vi "Shift.vi"(4 "Step count":i32, 5 "Step time (in ms)":u32, 6 "Absolute position":u16(ring) items=["Number of steps", "Absolute position"], 7 "Step size":i32, 8 "error in (no error)":errorcluster, 9 "Final position":i32, 10 "Movement direction":u16(ring) items=["Down", "Up", "Right", "Left"], 11 "Control in":refnum<vi>) -> (0 "error out":errorcluster, 3 "Current position":i32)   [LabVIEW 2019]
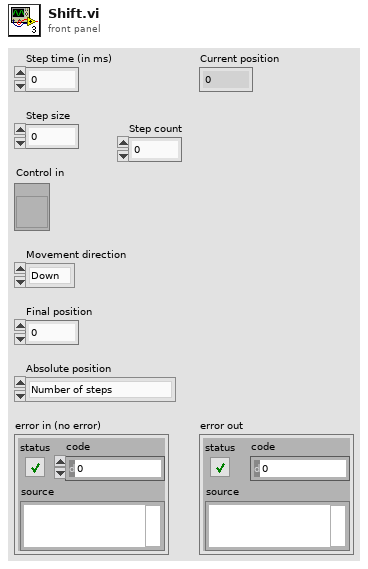
[diagram p1: front panel]
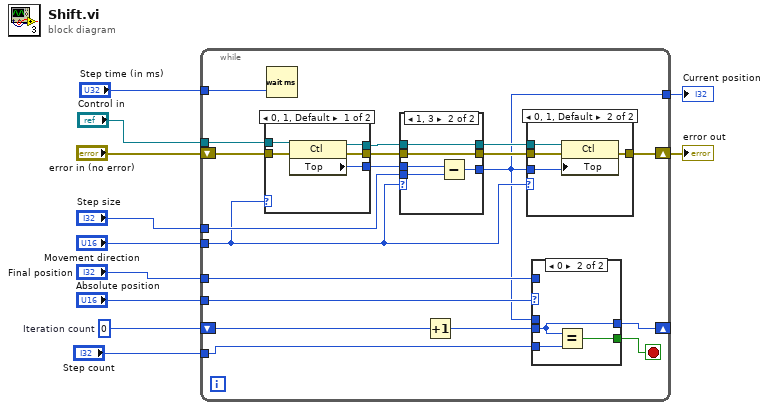
[diagram p0: block diagram]
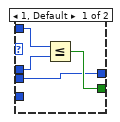
[diagram p2: hidden frame]
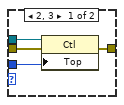
[diagram p3: hidden frame]
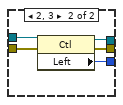
[diagram p4: hidden frame]
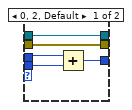
[diagram p5: hidden frame]
diagram:
  w2 = 0  # Iteration count
  n1 = while {
    tunnel: "Control in" -> [w30]
    tunnel: "Movement direction" -> [w26]
    tunnel: "Step size" -> [w27]
    tunnel: "Step time (in ms)" -> [w21]
    shift-right: [w20] -> w8
    shift-left: "error in (no error)" -> [w29]
    tunnel: "Absolute position" -> [w19]
    tunnel: [w17] -> w10
    tunnel: "Final position" -> [w18]
    shift-right: [w15] -> _
    shift-left: w2 -> [w14]
    tunnel: "Step count" -> [w12]
    stop <- w16 stop-if-true
    n2 = case shown="0, 1, Default" w26 {
      tunnel: w30 -> [w50 w55]
      tunnel: w29 -> [w49 w54]
      tunnel: [w48 w53] -> w28
      tunnel: [w47 w52] -> w25
      tunnel: [w46 w51] -> w22
      frame 0, 1, Default {
        n3 = property class="Ctl"(reference=w50, error in=w49) -> (reference out=w46:refnum<vi>, error out=w47:errorcluster, "Top"=w48:i32)
      }
      frame 2, 3 {
        n4 = property class="Ctl"(reference=w55, error in=w54) -> (reference out=w51:refnum<vi>, error out=w52:errorcluster, "Left"=w53:i32)
      }
    }
    n5 = Wait (ms)(milliseconds to wait=w21) -> ()  [unwired: 1 out]
    n6 = case shown="1, 3" w26 {
      tunnel: w28 -> [w60 w65]
      tunnel: [w59 w64] -> w17
      tunnel: w27 -> [w58 w63]
      tunnel: w25 -> [w57 w62]
      tunnel: [w57 w62] -> w24
      tunnel: [w56 w61] -> w23
      tunnel: w22 -> [w56 w61]
      frame 0, 2, Default {
        n7 = Add(x=w60, y=w58) -> (x+y=w59:i32)
      }
      frame 1, 3 {
        n8 = Subtract(x=w65, y=w63) -> (x-y=w64:i32)
      }
    }
    n9 = Increment(x=w14) -> (x+1=w13:i32)
    n10 = case shown="0, 1, Default" w26 {
      tunnel: w24 -> [w41 w45]
      tunnel: [w39 w44] -> w20
      tunnel: w23 -> [w40 w43]
      tunnel: w17 -> [w38 w42]
      frame 2, 3 {
        n11 = property class="Ctl"(reference=w40, error in=w41, "Top"=w38) -> (error out=w39:errorcluster)  [unwired: 1 out]
      }
      frame 0, 1, Default {
        n12 = property class="Ctl"(reference=w43, error in=w45, "Top"=w42) -> (error out=w44:errorcluster)  [unwired: 1 out]
      }
    }
    n13 = case shown="0" w19 {
      tunnel: w18 -> [w33 _]
      tunnel: w17 -> [w34 _]
      tunnel: [w32 w36] -> w16
      tunnel: w13 -> [w31 w35]
      tunnel: [w31 w35] -> w15
      tunnel: w12 -> [_ w37]
      frame 1, Default {
        n14 = Less Or Equal?(x=w33, y=w34) -> (x <= y?=w32:bool)
      }
      frame 0 {
        n15 = Equal?(x=w35, y=w37) -> (x = y?=w36:bool)
      }
    }
  }
  "error out" <- w8
  "Current position" <- w10
